vi "Filter Error Codes__jki_lib_error_handling -- VI Tester.vi"   [LabVIEW 2013]
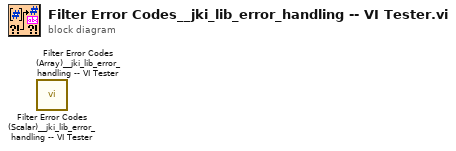
[diagram p0: block diagram]
diagram:
  n1 = call "Filter Error Codes (Scalar)__jki_lib_error_handling -- VI Tester.vi"() -> ()  [unwired: 9 in, 3 out]
  n2 = call "Filter Error Codes (Array)__jki_lib_error_handling -- VI Tester.vi"() -> ()  [unwired: 9 in, 3 out]
